vi "ResetBit(U32[] ).vi"(8 "error in (no error)":errorcluster caption="错误输入（无错误）", 10 "Bit(0-31)":u8[](array[numeric]), 11 "Input(U32)":u32 format="%.0x") -> (0 "error out":errorcluster caption="错误输出", 3 "Output(32)":u32 format="%.0b")   [LabVIEW 2012]
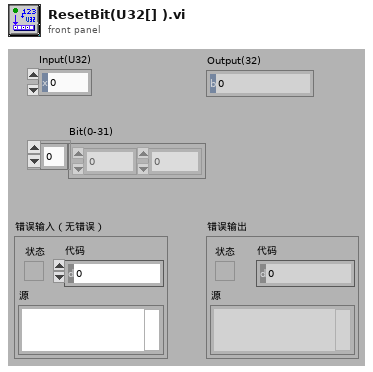
[diagram p1: front panel]
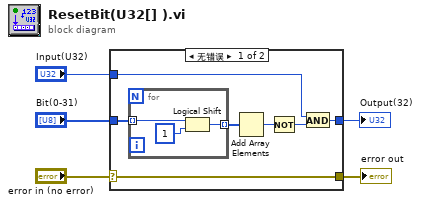
[diagram p0: block diagram]
diagram:
  n1 = case shown="无错误" "error in (no error)" {
    selector: "error in (no error)" -> [w12 w16]
    tunnel: [w12 w16] -> w4
    tunnel: "Input(U32)" -> [w11 _]
    tunnel: [w10 _] -> w2
    tunnel: "Bit(0-31)" -> [w8 _]
    frame No Error {
      n2 = for {
        tunnel: [w14] -> w7 mode=indexing
        tunnel: w8 -> [w13] mode=indexing
        n3 = Logical Shift(y=w13, x=u32 1) -> (x << y=w14:u32)
      }
      n4 = Add Array Elements(numeric array=w7) -> (sum=w6:u32)
      n5 = Not(x=w6) -> (.not. x?=w9:u32)
      n6 = And(x=w11, y=w9) -> (x .and. y?=w10:u32)
    }
    frame Error {
    }
  }
  "error out" <- w4
  "Output(32)" <- w2
